vi "SR430.constructor.vi"(0 "name":string, 2 "data in":string, 5 "error in (no error)":errorcluster) -> (14 "i ref out":refnum<vi>, 16 "data out":string, 19 "error out":errorcluster)   [LabVIEW 2014, in "SR430.lvlib"]
doc: "constructor of the SR430 class."
uses:
  SR430.lvlib
  CS_Core/CSApplicationBaseClasses/MCSBase/MCSBase.statusType.ctl
  CS_Core/CSApplicationBaseClasses/DeviceBase/DeviceBase.myEventNames.ctl
  CSlibraries/UtilityLib/UtilityLib.valueStatus.ctl
  CS_Core/CSSystem/CSSystemLib/CSSystemLib.lvlib
  instr.lib/SR430/SR430Driver.lvlib
  CS_Core/CSApplicationBaseClasses/DeviceBase/DeviceBase.lvlib
  CS_Core/CSApplicationBaseClasses/MCSBase/MCSBase.lvlib
  CSlibraries/UtilityLib/UtilityLib.lvlib
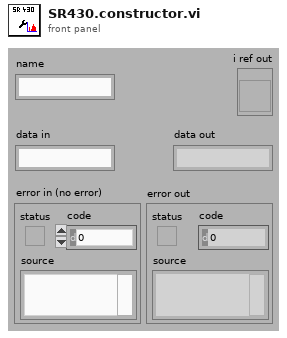
[diagram p1: front panel]
types:
  T1 = enum16{"SetAttribute", "GetAttribute", "CreateAttribute", "DestroyAttribute", "DestroyAllAtributes"}
  T2 = typedef "UtilityLib.lvlib/UtilityLib.valueStatus.ctl" = enum16{"no info available", "stand by/off", "on", "warning", "alarm/malfunction", "not implemented", "user action required", "important information", "system default", "control default", "indicator default", "button default"}
  T3 = typedef "DeviceBase.lvlib/DeviceBase.myEventNames.ctl" = enum16{"lvmsg://Initialize", "lvmsg://Close", "lvmsg://Configure", "lvmsg://Reset", "lvmsg://IDQuery"}
  T4 = typedef "MCSBase.lvlib/MCSBase.statusType.ctl" = i32
  T5 = typedef "SR430.lvlib/SR430.i attribute.ctl" = cluster{"initialized":bool, "SR430 VISA Cluster":T6}
  T6 = typedef "SR430Driver.lvlib/SR430_VISA Control.ctl" = cluster{"VISA resource name":refnum<visa-resource-name>}
  T7 = typedef "MCSBase.lvlib/MCSBase.i attribute.ctl" = cluster{"actValues":T8, "nomValues":T8}
  T8 = typedef "MCSBase.lvlib/MCSBase.parameters.ctl" = cluster{"counts":i32, "totalCounts":i32, "status":i32, "binWidth [us]":dbl, "nOfBins":i32, "nOfRecords":i32, "discLevel [V]":dbl, "discSlope":bool, "triggerLevel [V]":dbl, "triggerSlope":bool, "serviceIDs":cluster{"countslID":i32, "totalCountsID":i32, "binWidthID":i32, "nOfBinsID":i32, "nOfRecordsID":i32, "statusID":i32, "discLevelID":i32, "discSlopeID":i32, "triggerLevelID":i32, "triggerSlopeID":i32}}
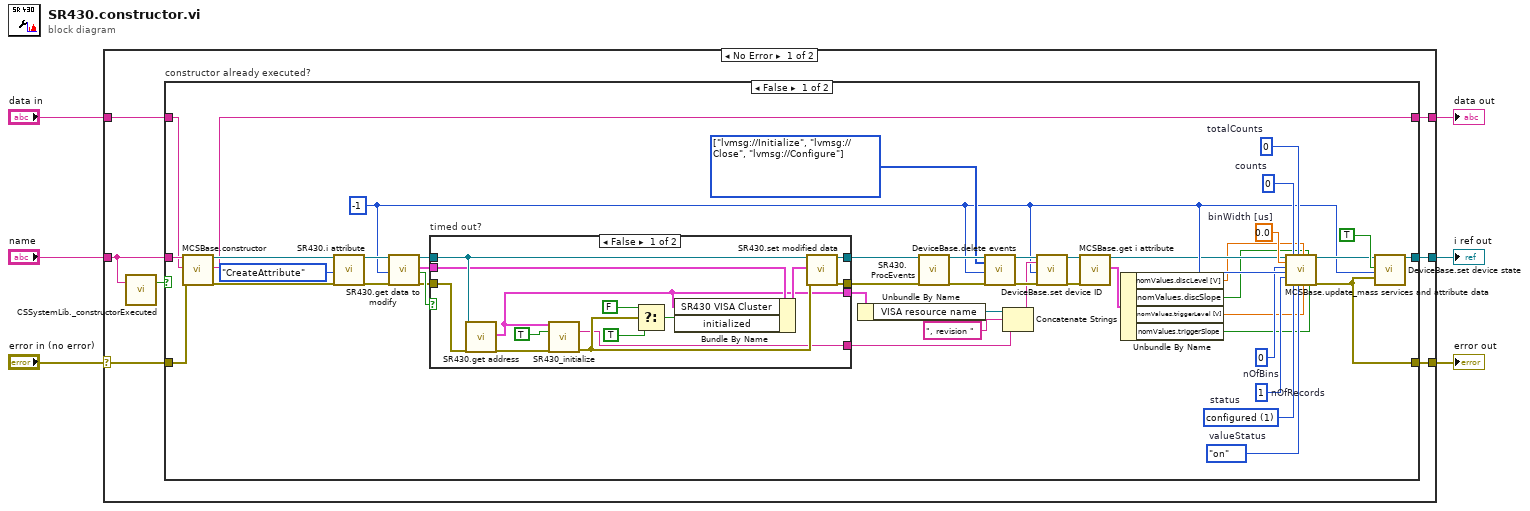
[diagram p0: block diagram]
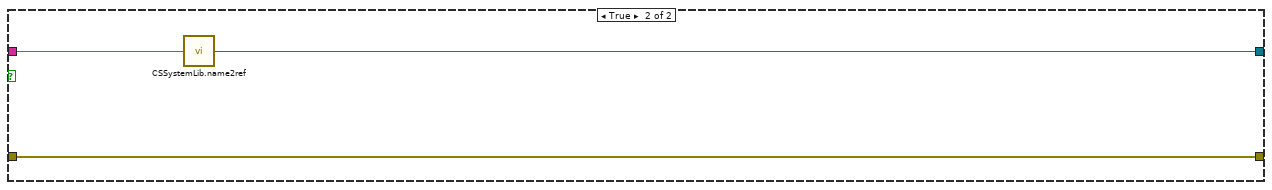
[diagram p3: hidden frame]
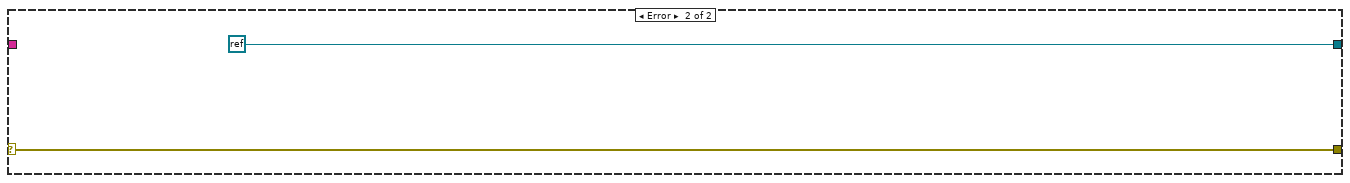
[diagram p4: hidden frame]
diagram:
  n1 = case shown="No Error" "error in (no error)" {
    selector: "error in (no error)" -> [w11 w78]
    tunnel: "name" -> [w10 _]
    tunnel: [w13 refnum<k0> refnum ("Not a Refnum Constant")] -> w5
    tunnel: [w12 w78] -> w4
    tunnel: "data in" -> [w8 _]
    tunnel: [w7 _] -> w1
    frame No Error {
      n2 = call "CSSystemLib._constructorExecuted.vi"("name"=w10) -> ("constructor executed?"=w9:bool)  [unwired: 18 in]
      n3 = case "constructor already executed?" shown="False" w9 {
        tunnel: [w33 w76] -> w13
        tunnel: [w25 w75] -> w12
        tunnel: w11 -> [w55 w75]
        tunnel: w10 -> [w54 w77]
        tunnel: w8 -> [w53 _]
        tunnel: [w14 _] -> w7
        frame False {
          w23 = 0.0  # binWidth [us]
          w28 = UtilityLib.valueStatus."on"  # valueStatus
          w42 = T3[] [enum."lvmsg://Initialize", enum."lvmsg://Close", enum."lvmsg://Configure"] items=["lvmsg://Initialize", "lvmsg://Close", "lvmsg://Configure", "lvmsg://Reset", "lvmsg://IDQuery"] ("events")
          w22 = 0  # nOfBins
          w32 = T4 1 items=["unknown"=0, "configured"=1, "error"=32]  # status
          w29 = 1  # nOfRecords
          w30 = 0  # totalCounts
          w31 = 0  # counts
          w24 = -1 ("ms timeout (10000)")
          n4 = call "MCSBase.constructor.vi"("name"=w54, "data in"=w53, "error in (no error)"=w55) -> ("i ref out"=w58:refnum<vi>, "data out"=w14:string, "error out"=w57:errorcluster)  [unwired: 14 in]
          n5 = call "SR430.i attribute.vi"("VI Refnum"=w58, "Action"=T1."CreateAttribute", "error in (no error)"=w57) -> ("VI Refnum out"=w52:refnum<vi>, "error out"=w51:errorcluster)  [unwired: 14 in, 1 out]
          n6 = call "SR430.get data to modify.vi"("i ref in"=w52, "ms timeout (10000)"=w24, "error in (no error)"=w51) -> ("i ref out"=w47:refnum<vi>, "i attribute"=w45:T5, "timed out"=w50:bool, "error out"=w46:errorcluster)  [unwired: 13 in]
          n7 = case "timed out?" shown="False" w50 {
            tunnel: [w72 w74] -> w49
            tunnel: [w71 w73] -> w48
            tunnel: w47 -> [w68 w74]
            tunnel: w46 -> [w70 w73]
            tunnel: w45 -> [w61 _]
            tunnel: [w60 _] -> w36
            tunnel: [w59 _] -> w39
            frame False {
              n8 = call "SR430.get address.vi"("i ref in"=w68, "error in (no error)"=w70) -> ("address"=w59:T6, "error out"=w67:errorcluster)  [unwired: 15 in, 1 out]
              n9 = call "SR430_initialize.vi"("SR430 VISA Cluster"=w59, "Revision Query (F: Check)"=TRUE, "error in (no error)"=w67) -> ("Revision"=w60:string, "error out"=w62:errorcluster)  [unwired: 9 in, 2 out]
              n10 = Select(t=FALSE, s=w62, f=TRUE) -> (s? t:f=w63:bool)
              n11 = Bundle By Name(cluster=w61, "SR430 VISA Cluster"=w59, "initialized"=w63) -> (w69:T5)
              n12 = call "SR430.set modified data.vi"("i ref in"=w68, "i attribute"=w69, "error in (no error)"=w62) -> ("i ref out"=w72:refnum<vi>, "error out"=w71:errorcluster)  [unwired: 15 in]
            }
            frame True {
            }
          }
          n13 = Unbundle By Name(w39) -> ("VISA resource name"=w38:refnum<visa-resource-name>)
          n14 = call "SR430.ProcEvents.vi"("i ref in"=w49, "error in (no error)"=w48) -> ("i ref out"=w44:refnum<vi>, "error out"=w43:errorcluster)  [unwired: 16 in]
          n15 = call "DeviceBase.delete events.vi"("i ref in"=w44, "events"=w42, "ms timeout (10000)"=w24, "error in (no error)"=w43) -> ("i ref out"=w41:refnum<vi>, "error out"=w40:errorcluster)  [unwired: 13 in, 1 out]
          n16 = Concatenate Strings(w38, ", revision " ("string"), w36) -> (w35:string)
          n17 = call "DeviceBase.set device ID.vi"("i ref in"=w41, "deviceID"=w35, "ms timeout (10000)"=w24, "error in (no error)"=w40) -> ("i ref out"=w27:refnum<vi>, "error out"=w20:errorcluster)  [unwired: 13 in, 1 out]
          n18 = call "MCSBase.get i attribute.vi"("i ref in"=w27, "error in (no error)"=w20) -> ("i ref out"=w21:refnum<vi>, "i attribute"=w19:T7)  [unwired: 15 in, 1 out]
          n19 = Unbundle By Name(w19) -> ("nomValues.discLevel [V]"=w18:dbl, "nomValues.discSlope"=w17:bool, "nomValues.triggerLevel [V]"=w16:dbl, "nomValues.triggerSlope"=w15:bool)
          n20 = call "MCSBase.update_mass services and attribute data.vi"("i ref in"=w21, "binWidth [us]"=w23, "nOfBins"=w22, "ms timeout (10000)"=w24, "nOfRecords"=w29, "counts"=w31, "status"=w32, "totalCounts"=w30, "valueStatus"=w28, "discLevel [V]"=w18, "triggerLevel [V]"=w16, "discSlope"=w17, "triggerSlope"=w15) -> ("i ref out"=w26:refnum<vi>, "error out"=w25:errorcluster)  [unwired: 4 in, 1 out]
          n21 = call "DeviceBase.set device state.vi"("i ref in"=w26, "implicit"=TRUE, "ms timeout (10000)"=w24, "device error"=w25) -> ("i ref out"=w33:refnum<vi>)  [unwired: 13 in, 2 out]
        }
        frame True {
          n22 = call "CSSystemLib.name2ref.vi"("name"=w77) -> ("obj refnum"=w76:refnum<vi>)
        }
      }
    }
    frame Error {
    }
  }
  "i ref out" <- w5
  "error out" <- w4
  "data out" <- w1
